vi "Output_v00.vi"(8 "Outputs":T2, 11 "Safety First":T1) -> ()   [LabVIEW 2010]
doc: "Outputs the signals to FPGA output nodes, after a variable rate-limiter has been applied."
uses:
  Strict Type Defs/Safety First.ctl
  <vilib>/rvi/Analysis/common/polyVINode/niFpgaPolyViWrapper.xnode
  <vilib>/eio/EIONode/EIONode.xnode
  <vilib>/rvi/eio/nirviEIOImplementation/nirviEIOImplementation.xnode
  <vilib>/rvi/eio/common/nirviEmuClasses.ctl
  <vilib>/express/rvi/analysis/control/nonlinear/niFPGA Rate Limiter.vi
  <vilib>/express/rvi/analysis/control/nonlinear/niFPGA Rate Limiter (I16).vi
  <vilib>/rvi/eio/common/nirviEmuTemplateMethod_noerrors.vi
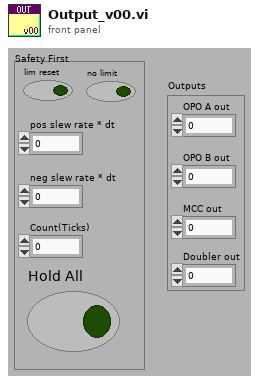
[diagram p1: front panel]
types:
  T1 = typedef "Safety First.ctl" = cluster{"lim reset":bool, "no limit":bool, "pos slew rate * dt":i16, "neg slew rate * dt":i16, "Hold All":bool, "Count(Ticks)":u32}
  T2 = cluster{"OPO A out":i16, "OPO B out":i16, "MCC out":i16, "Doubler out":i16}
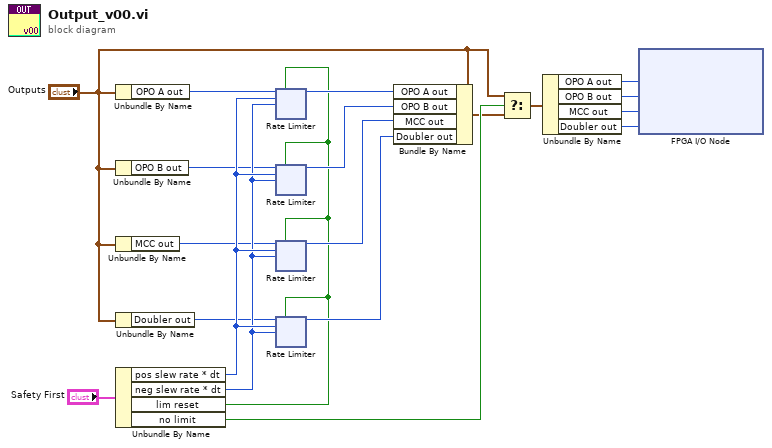
[diagram p0: block diagram]
diagram:
  n1 = Unbundle By Name("Outputs") -> ("OPO A out"=w19:i16)
  n2 = Unbundle By Name("Outputs") -> ("OPO B out"=w16:i16)
  n3 = Unbundle By Name("Outputs") -> ("MCC out"=w15:i16)
  n4 = Unbundle By Name("Outputs") -> ("Doubler out"=w14:i16)
  n5 = Unbundle By Name("Safety First") -> ("pos slew rate * dt"=w18:i16, "neg slew rate * dt"=w17:i16, "lim reset"=w8:bool, "no limit"=w9:bool)
  n6 = xnode "Rate Limiter"("pos slew rate * dt"=w18, "input"=w19, "neg slew rate * dt"=w17, "reset"=w8) -> ("output"=w13:i16)
  n7 = xnode "Rate Limiter"("pos slew rate * dt"=w18, "input"=w16, "neg slew rate * dt"=w17, "reset"=w8) -> ("output"=w12:i16)
  n8 = xnode "Rate Limiter"("pos slew rate * dt"=w18, "input"=w15, "neg slew rate * dt"=w17, "reset"=w8) -> ("output"=w11:i16)
  n9 = xnode "Rate Limiter"("pos slew rate * dt"=w18, "input"=w14, "neg slew rate * dt"=w17, "reset"=w8) -> ("output"=w10:i16)
  n10 = Bundle By Name(cluster="Outputs", "OPO A out"=w13, "OPO B out"=w12, "MCC out"=w11, "Doubler out"=w10) -> (w2:T2)
  n11 = Select(t="Outputs", s=w9, f=w2) -> (s? t:f=w7:T2)
  n12 = Unbundle By Name(w7) -> ("OPO A out"=w6:i16, "OPO B out"=w5:i16, "MCC out"=w4:i16, "Doubler out"=w3:i16)
  n13 = xnode "FPGA I/O Node"("Connector0/AO0"=w6, "Connector0/AO1"=w5, "Connector0/AO2"=w4, "Connector0/AO3"=w3) -> ()  [unwired: 4 in, 4 out]
